vi "Save Image To File (Core).vi"(7 "Save Format":T1, 8 "error in (no error)":errorcluster, 10 "Picture":T2, 11 "Path In":string) -> (0 "error out":errorcluster, 3 "Path Out":string)   [LabVIEW 2020, in "G-Image.lvlib"]
doc: "Retrieve audio file information. Some codecs (mp3) require the entire file be parsed to accurately determine the length, which can take time for very large files.\n\nSupported codecs: flac, mp3, ogg (vorbis), and wav."
uses:
  G-Image.lvlib
  <vilib>/picture/picture.llb/imagedata.ctl
  Controls/Image Save Format.ctl
  Private/ARGB To RGBA.vi
  <vilib>/Utility/error.llb/Error Cluster From Error Code.vi
  lib/g_image_32.dll
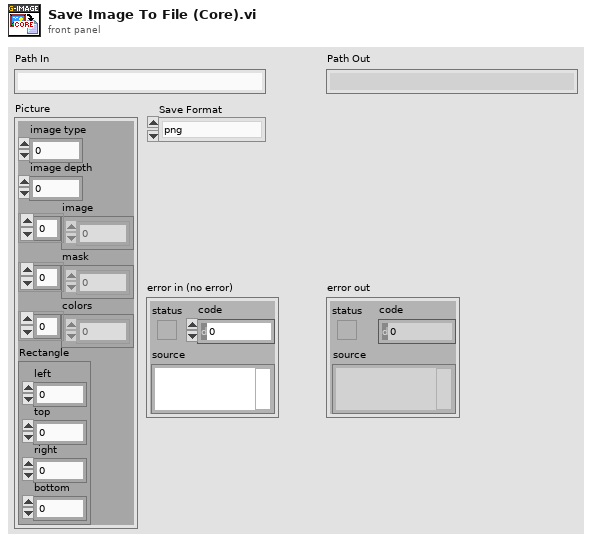
[diagram p1: front panel]
types:
  T1 = typedef "G-Image.lvlib/Image Save Format.ctl" = enum16{"png", "jpg", "bmp", "gif", "tga"}
  T2 = typedef "imagedata.ctl" = cluster{"image type":i32, "image depth":i32, "image":u8[], "mask":u8[], "colors":u32[], "Rectangle":cluster{"left":i16, "top":i16, "right":i16, "bottom":i16}}
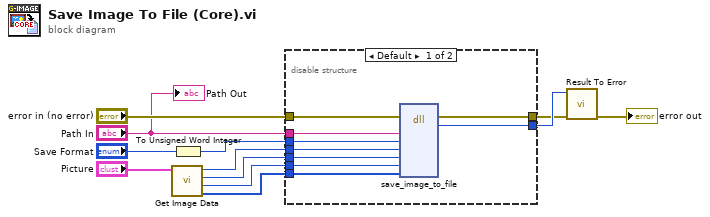
[diagram p0: block diagram]
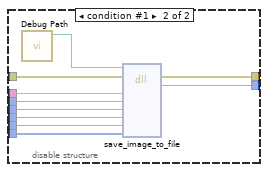
[diagram p2: hidden frame]
diagram:
  n1 = call "Get Image Data.vi"("Image"="Picture") -> ("Image (RGBA)"=w1:u8[], "Channels"=w2:i32, "Height"=w3:i32, "Width"=w4:i32)  [unwired: 7 in]
  n2 = To Unsigned Word Integer(number="Save Format") -> (unsigned 16bit integer=w7:u16)
  n3 = disable-structure shown="Default" {
    disable-tunnel: [w21 w31] -> w10
    disable-tunnel: "error in (no error)" -> [w20 w30]
    disable-tunnel: "Path In" -> [w19 w29]
    disable-tunnel: [w18 w28] -> w11
    disable-tunnel: w7 -> [w17 w27]
    disable-tunnel: w4 -> [w16 w26]
    disable-tunnel: w3 -> [w15 w25]
    disable-tunnel: w2 -> [w14 w24]
    disable-tunnel: w1 -> [w13 w23]
    frame condition #0 (active) {
      n4 = dll-call lib="C:/github/dataflowg/g-image/src/LabVIEW/G-Image/lib/g_image_*.*" fn="save_image_to_file"(error in=w20, "file_name"=w19, "format"=w17, "width"=w16, "height"=w15, "channels"=w14, "image_data"=w13) -> (error out=w21:errorcluster, "result"=w18:i32)  [unwired: 8 in, 1 out]
    }
    frame condition #1 {
      n5 = call "Debug Path.vi"() -> ("Debug Path"=w22:path)  [unwired: 11 in]
      n6 = dll-call lib="?" fn="save_image_to_file"(path in=w22, error in=w30, "file_name"=w29, "format"=w27, "width"=w26, "height"=w25, "channels"=w24, "image_data"=w23) -> (error out=w31:errorcluster, "result"=w28:i32)  [unwired: 7 in, 1 out]
    }
  }
  n7 = call "Result To Error.vi"("error in (no error)"=w10, "Result Code"=w11) -> ("error out"=→"error out":errorcluster)  [unwired: 9 in]
  "Path Out" <- "Path In"
